vi "sort input and output channels.vi"(11 "Channels In":T1[](array[typedef])) -> (2 "Outputs":T1[](array[typedef]), 3 "Inputs":T1[](array[typedef]))   [LabVIEW 2015]
uses:
  Shared/Controls/Data Model/Channel.ctl
  SubVIs/Modbus Type.ctl
  <vilib>/NI Veristand/Custom Device API/Custom Device Channel Type.ctl
  Shared/Controls/Data Model/Mapping.ctl
  Shared/Controls/Data Model/DataType.ctl
  <vilib>/NI Veristand/Custom Device API/Custom Device Item Ref.ctl
  <vilib>/NI VeriStand/Custom Device API/Custom Device API.lvlib
  Shared/Modbus Master Shared.lvlib
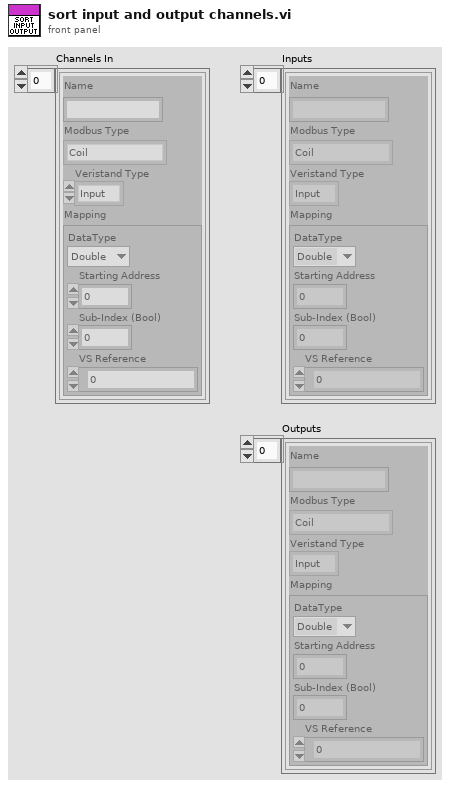
[diagram p1: front panel]
types:
  T1 = typedef "Modbus Master Shared.lvlib/Channel.ctl" = cluster{"Name":string, "Modbus Type":T2, "Veristand Type":T3, "Mapping":T4}
  T2 = typedef "Modbus Master Shared.lvlib/Modbus Type.ctl" = enum16{"Coil", "Discrete Input", "Holding Register", "Input Register"}
  T3 = typedef "Custom Device API.lvlib/Custom Device Channel Type.ctl" = enum16{"Input", "Output"}
  T4 = typedef "Modbus Master Shared.lvlib/Mapping.ctl" = cluster{"DataType":T5, "Starting Address":u16, "Sub-Index (Bool)":u16, "VS Reference":T6}
  T5 = typedef "Modbus Master Shared.lvlib/DataType.ctl" = enum16{"Double", "Single", "I64", "I32", "I16", "I8", "U64", "U32", "U16", "U8", "Boolean"}
  T6 = typedef "Custom Device API.lvlib/Custom Device Item Ref.ctl" = u64
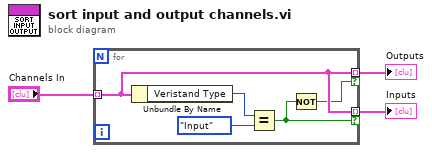
[diagram p0: block diagram]
diagram:
  n1 = for {
    tunnel: "Channels In" -> [w6] mode=indexing
    tunnel: [w6] -> w2 mode=indexing if=w5
    tunnel: [w6] -> w3 mode=indexing if=w4
    n2 = Unbundle By Name(w6) -> ("Veristand Type"=w8:T3)
    n3 = Equal?(x=w8, y=Custom_Device_Channel_Type."Input") -> (x = y?=w5:bool)
    n4 = Not(x=w5) -> (.not. x?=w4:bool)
  }
  "Outputs" <- w3
  "Inputs" <- w2
